vi "RF_SPW_Upsample.vi"(7 "Header In":T1={"header info"={"Header"="", "Head length"=0}, "A/D info"={"# rf points per line"=0, "# lines per scan"=0, "sample rate MHz"=0, "# A/D bits"=0, "# bytes per A/D"=0, "TGC Flag"=0, "A/D Type"=""}, "Tranducer Info"={"bandwidth"=0.0, "center freq"=0.0, "start freq"=0.0, "ID"=0}, "Scan Info"={"delay"=0.0, "pivot distance"=0.0, "sector scan angle"=0.0, "operator"="", "Scan Mode"="", "location"=""}, "Time/Date Info"={"date"="", "time"=""}, "RF Info"={"RF file name"="", "RF file att"="", "RF cal file name"="", "RF cal file att"=""}, "Patient Info"={"ID"="", "extended ID"="", "age"=0, "sex"="", "previously\nscanned"="", "PSA"=0.0, "LOS"=1, "Ethnicty 2"=3, "Race"=3}, "Tissue Type"={"organ"=0, "disease type"=0, "disease location"=0, "IQ_pts"=0, "RcvBuffer"=0, "RcvFrame"=0, "IQBuff"=0, "IQFrame"=0, "IQPage"=0}, "Votage scaling"={"Digitizer (dB)"=0.0, "Gain (dB)"=0.0, "Atten (dB)"=0.0}, "Comment"="", "Misc Info"={"avg num"=0, "c speed"=0, "Div By or SF zones"=0, "XMIT CHS"=0, "RCV CHS"=0, "Xmit angle"=0.0}, "Therapy Parameters"={"Theraputic Freq (MHz)"=0.1, "Time on (s)"=1.0, "Therapy amplitude (mV)"=50.0, "Lines Before"=20, "Lines After"=80}, "Scan Settings"={"Energy (uJ or V)"=0, "Damp (Ohm) or Fc"=0, "HP Filt (KHz)"=0, "LP Filt (MHz)"=0, "Gain (db)"=0, "prf (kHz)"=0.0, "Distance between\nscan lines (um)"=0, "Distance between\nscan planes (um)"=0, "Scan line gap (um)"=0.0, "Scan plane gap (um)"=0.0}, "Compression Parameters"={"F1 (MHz)"=0.0, "F2 (MHz)"=0.0, "% taper"=0.0, "duration"=0.0}, "Patient Info Xtra"={"First Name"="", "Last Name"="", "Notes"=""}, "ROI Box"=[]} {"Compression Parameters"."% taper" min=50 max=1000 format="%.2f"; "Compression Parameters"."F2 (MHz)" format="%.3f"; "Compression Parameters"."F1 (MHz)" format="%.3f"; "Scan Settings"."prf (kHz)" format="%.2f"; "Therapy Parameters"."Therapy amplitude (mV)" min=50 max=1000 format="%.2f"; "Therapy Parameters"."Time on (s)" format="%.3f"; "Therapy Parameters"."Theraputic Freq (MHz)" format="%.3f"; "Patient Info"."Race" items=["Am Ind or Alaska", "Asian", "Hawaiian, Pac Isl", "Black or Afr Amer", "White", "more than one race", "unknown"]; "Patient Info"."Ethnicty 2" items=["Hispanic", "Non-Hispanic", "unknown"]; "Patient Info"."LOS" items=["1", "2", "3", "4", "5"]; "Patient Info"."PSA" format="%.1f"; "Scan Info"."delay" format="%.2f"; "Scan Info"."pivot distance" format="%.2f"; "Scan Info"."sector scan angle" format="%.2f"; "Tranducer Info"."bandwidth" format="%.2f"; "Tranducer Info"."center freq" format="%.2f"; "Tranducer Info"."start freq" format="%.2f"}, 9 "RF Data In":i16[](array[numeric])) -> (0 "Header Out":T1={"header info"={"Header"="", "Head length"=0}, "A/D info"={"# rf points per line"=0, "# lines per scan"=0, "sample rate MHz"=0, "# A/D bits"=0, "# bytes per A/D"=0, "TGC Flag"=0, "A/D Type"=""}, "Tranducer Info"={"bandwidth"=0.0, "center freq"=0.0, "start freq"=0.0, "ID"=0}, "Scan Info"={"delay"=0.0, "pivot distance"=0.0, "sector scan angle"=0.0, "operator"="", "Scan Mode"="", "location"=""}, "Time/Date Info"={"date"="", "time"=""}, "RF Info"={"RF file name"="", "RF file att"="", "RF cal file name"="", "RF cal file att"=""}, "Patient Info"={"ID"="", "extended ID"="", "age"=0, "sex"="", "previously\nscanned"="", "PSA"=0.0, "LOS"=1, "Ethnicty 2"=3, "Race"=3}, "Tissue Type"={"organ"=0, "disease type"=0, "disease location"=0, "IQ_pts"=0, "RcvBuffer"=0, "RcvFrame"=0, "IQBuff"=0, "IQFrame"=0, "IQPage"=0}, "Votage scaling"={"Digitizer (dB)"=0.0, "Gain (dB)"=0.0, "Atten (dB)"=0.0}, "Comment"="", "Misc Info"={"avg num"=0, "c speed"=0, "Div By or SF zones"=0, "XMIT CHS"=0, "RCV CHS"=0, "Xmit angle"=0.0}, "Therapy Parameters"={"Theraputic Freq (MHz)"=0.0, "Time on (s)"=0.0, "Therapy amplitude (mV)"=0.0, "Lines Before"=0, "Lines After"=0}, "Scan Settings"={"Energy (uJ or V)"=0, "Damp (Ohm) or Fc"=0, "HP Filt (KHz)"=0, "LP Filt (MHz)"=0, "Gain (db)"=0, "prf (kHz)"=0.0, "Distance between\nscan lines (um)"=0, "Distance between\nscan planes (um)"=0, "Scan line gap (um)"=0.0, "Scan plane gap (um)"=0.0}, "Compression Parameters"={"F1 (MHz)"=0.0, "F2 (MHz)"=0.0, "% taper"=0.0, "duration"=0.0}, "Patient Info Xtra"={"First Name"="", "Last Name"="", "Notes"=""}, "ROI Box"=[0, 0, 0, 0]} {"Compression Parameters"."% taper" min=50 max=1000 format="%.2f"; "Compression Parameters"."F2 (MHz)" format="%.3f"; "Compression Parameters"."F1 (MHz)" format="%.3f"; "Scan Settings"."prf (kHz)" format="%.2f"; "Therapy Parameters"."Therapy amplitude (mV)" min=50 max=1000 format="%.2f"; "Therapy Parameters"."Time on (s)" format="%.3f"; "Therapy Parameters"."Theraputic Freq (MHz)" format="%.3f"; "Patient Info"."Race" items=["Am Ind or Alaska", "Asian", "Hawaiian, Pac Isl", "Black or Afr Amer", "White", "more than one race", "unknown"]; "Patient Info"."Ethnicty 2" items=["Hispanic", "Non-Hispanic", "unknown"]; "Patient Info"."LOS" items=["1", "2", "3", "4", "5"]; "Patient Info"."PSA" format="%.1f"; "Scan Info"."delay" format="%.2f"; "Scan Info"."pivot distance" format="%.2f"; "Scan Info"."sector scan angle" format="%.2f"; "Tranducer Info"."bandwidth" format="%.2f"; "Tranducer Info"."center freq" format="%.2f"; "Tranducer Info"."start freq" format="%.2f"}, 1 "RF Out 2D":i16[][](graph), 2 "RF pts out":i32, 3 "RF Array Out":i16[](array[numeric]))   [LabVIEW 2022 SP3]
uses:
  ViewData/-ReadEye/Header.ctl
  <vilib>/Analysis/1siggen.llb/Ramp Pattern by Samples.vi
  <vilib>/gmath/NI_Gmath.lvlib
  <vilib>/Analysis/NI_AALBase.lvlib
panel:
  out "RF 2D in":i16[][](graph)
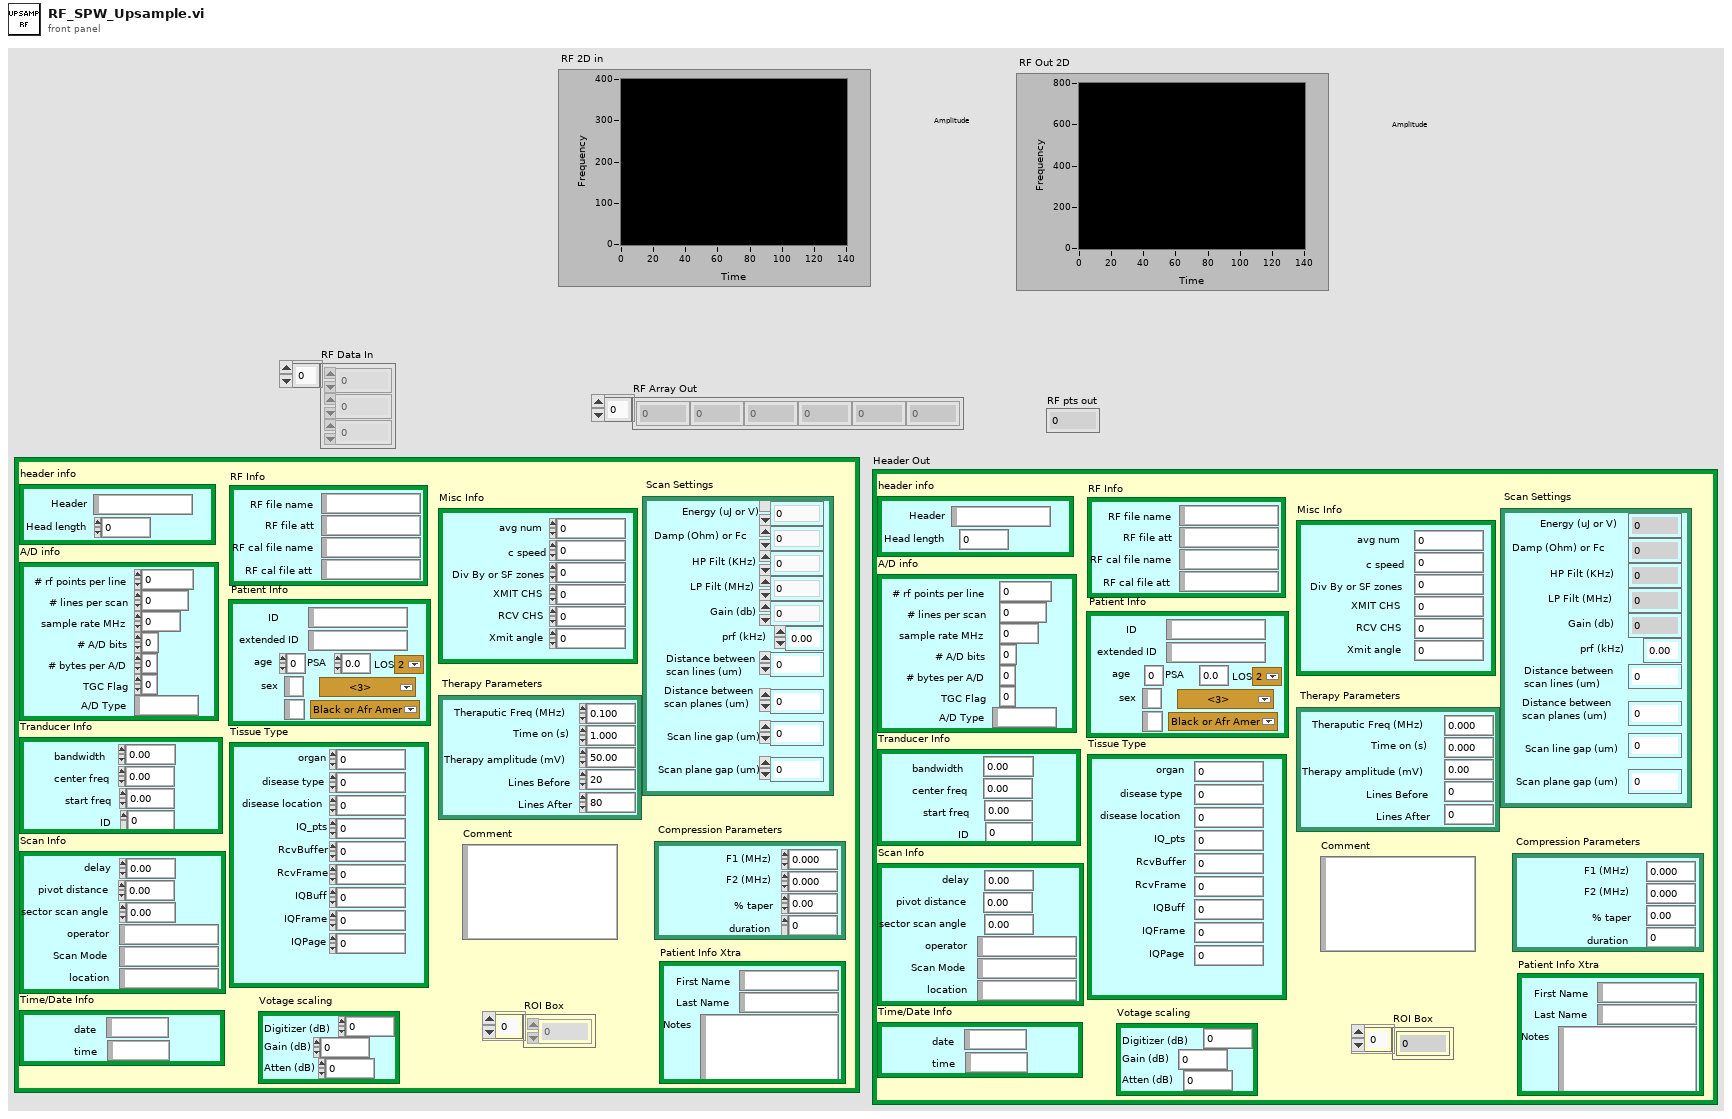
[diagram p1: front panel]
types:
  T1 = typedef "Header.ctl" = cluster{"header info":cluster{"Header":string, "Head length":i16}, "A/D info":cluster{"# rf points per line":u16, "# lines per scan":u16, "sample rate MHz":u16, "# A/D bits":i16, "# bytes per A/D":u16, "TGC Flag":u16, "A/D Type":string}, "Tranducer Info":cluster{"bandwidth":sgl, "center freq":sgl, "start freq":sgl, "ID":i32}, "Scan Info":cluster{"delay":sgl, "pivot distance":sgl, "sector scan angle":sgl, "operator":string, "Scan Mode":string, "location":string}, "Time/Date Info":cluster{"date":string, "time":string}, "RF Info":cluster{"RF file name":string, "RF file att":string, "RF cal file name":string, "RF cal file att":string}, "Patient Info":cluster{"ID":string, "extended ID":string, "age":u16, "sex":string, "previously\nscanned":string, "PSA":sgl, "LOS":u8, "Ethnicty 2":u8, "Race":u8}, "Tissue Type":cluster{"organ":i16, "disease type":i16, "disease location":i16, "IQ_pts":u16, "RcvBuffer":u8, "RcvFrame":u16, "IQBuff":u8, "IQFrame":u16, "IQPage":u8}, "Votage scaling":cluster{"Digitizer (dB)":sgl, "Gain (dB)":sgl, "Atten (dB)":sgl}, "Comment":string, "Misc Info":cluster{"avg num":u16, "c speed":i16, "Div By or SF zones":i16, "XMIT CHS":u8, "RCV CHS":u8, "Xmit angle":sgl}, "Therapy Parameters":cluster{"Theraputic Freq (MHz)":sgl, "Time on (s)":sgl, "Therapy amplitude (mV)":sgl, "Lines Before":u16, "Lines After":u16}, "Scan Settings":cluster{"Energy (uJ or V)":u8, "Damp (Ohm) or Fc":u8, "HP Filt (KHz)":u8, "LP Filt (MHz)":u8, "Gain (db)":u8, "prf (kHz)":sgl, "Distance between\nscan lines (um)":u16, "Distance between\nscan planes (um)":u16, "Scan line gap (um)":sgl, "Scan plane gap (um)":sgl}, "Compression Parameters":cluster{"F1 (MHz)":sgl, "F2 (MHz)":sgl, "% taper":sgl, "duration":sgl}, "Patient Info Xtra":cluster{"First Name":string, "Last Name":string, "Notes":string}, "ROI Box":u16[]}
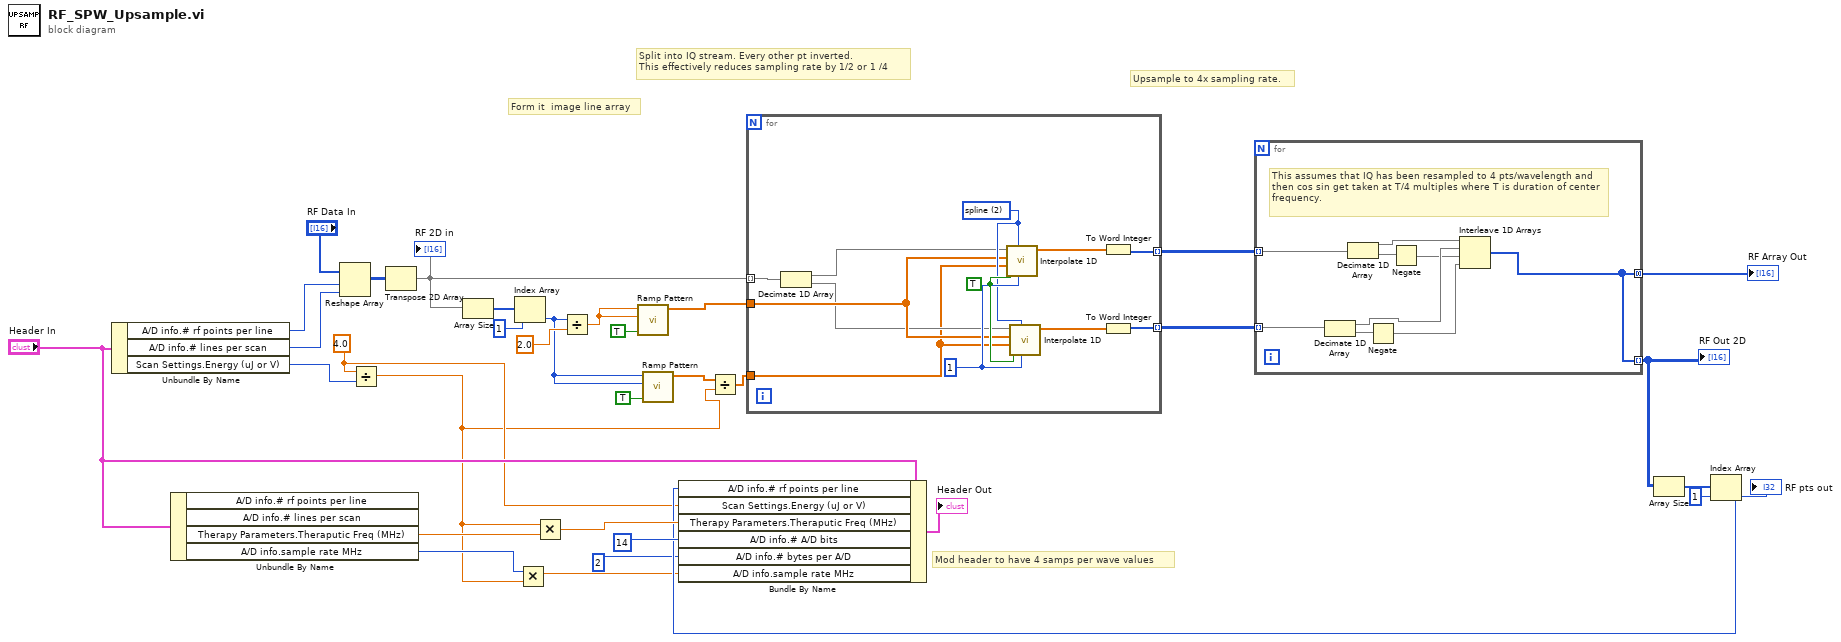
[diagram p0: block diagram]
diagram:
  w2 = sgl 4.0 ("value")
  # "Mod header to have 4 samps per wave values"
  # "Upsample to 4x sampling rate."
  # "Form it  image line array"
  # "Split into IQ stream. Every other pt inverted.\nThis effectively reduces sampling rate by 1/2 or 1 /4"
  n1 = Unbundle By Name("Header In") -> ("A/D info.# rf points per line"=w26:u16, "A/D info.# lines per scan"=w27:u16, "Scan Settings.Energy (uJ or V)"=w33:u8)
  n2 = Unbundle By Name("Header In") -> ("Therapy Parameters.Theraputic Freq (MHz)"=w31:sgl, "A/D info.sample rate MHz"=w4:u16)  [unwired: 2 out]
  n3 = Reshape Array("RF Data In", w26, w27) -> (w28:i16[][])
  n4 = Divide(x=w2, y=w33) -> (x/y=w1:sgl)
  n5 = Transpose 2D Array(2D array=w28) -> (transposed array=w16:i16[][])
  "RF 2D in" <- w16
  n6 = Array Size(array=w16) -> (size(s)=w23:i32[])
  n7 = Index Array(array=w23, index=1) -> (element=w8:i32)
  n8 = Multiply(x=w4, y=w1) -> (x*y=w3:sgl)
  n9 = Multiply(x=w1, y=w31) -> (x*y=w30:sgl)
  n10 = Divide(x=w8, y=sgl 2.0 ("value")) -> (x/y=w19:sgl)
  n11 = call-poly <vilib>:"Ramp Pattern.vi"("exclude end?"=TRUE, "end"=w19, "samples"=w19) -> ("Ramp Pattern"=w17:dbl[])  [unwired: 7 in, 1 out]
  n12 = call-poly <vilib>:"Ramp Pattern.vi"("exclude end?"=TRUE, "end"=w8, "samples"=w8) -> ("Ramp Pattern"=w7:dbl[])  [unwired: 7 in, 1 out]
  n13 = Divide(x=w7, y=w1) -> (x/y=w6:dbl[])
  n14 = for {
    tunnel: [w44] -> w25 mode=indexing
    tunnel: [w45] -> w24 mode=indexing
    tunnel: w16 -> [w35] mode=indexing
    tunnel: w17 -> [w40]
    tunnel: w6 -> [w34]
    w43 = 1 ("ntimes")
    w42 = TRUE ("X is monotonic")
    w41 = 2 items=["nearest", "linear", "spline", "cubic Hermite", "Lagrange"] ("method")
    n15 = Decimate 1D Array(w35) -> (w39:i16[], w38:i16[])
    n16 = call <vilib>:"Interpolate 1D.vi"("ntimes"=w43, "method"=w41, "X is monotonic"=w42, "xi"=w34, "X"=w40, "Y"=w39) -> ("yi"=w37:dbl[])  [unwired: 3 in, 2 out]
    n17 = call <vilib>:"Interpolate 1D.vi"("ntimes"=w43, "method"=w41, "X is monotonic"=w42, "xi"=w34, "X"=w40, "Y"=w38) -> ("yi"=w36:dbl[])  [unwired: 3 in, 2 out]
    n18 = To Word Integer(number=w37) -> (16bit integer=w44:i16[])
    n19 = To Word Integer(number=w36) -> (16bit integer=w45:i16[])
  }
  n20 = for {
    tunnel: [w46] -> w18 mode=concatenating
    tunnel: w25 -> [w54] mode=indexing
    tunnel: w24 -> [w53] mode=indexing
    tunnel: [w46] -> w15 mode=indexing
    # "This assumes that IQ has been resampled to 4 pts/wavelength and then cos sin get taken at T/4 multiples where T is duration of center frequency."
    n21 = Decimate 1D Array(w53) -> (w49:i16[], w51:i16[])
    n22 = Decimate 1D Array(w54) -> (w50:i16[], w52:i16[])
    n23 = Negate(x=w51) -> (-x=w47:i16[])
    n24 = Negate(x=w52) -> (-x=w48:i16[])
    n25 = Interleave 1D Arrays(w50, w49, w48, w47) -> (w46:i16[])
  }
  "RF Array Out" <- w18
  "RF Out 2D" <- w15
  n26 = Array Size(array=w15) -> (size(s)=w14:i32[])
  n27 = Index Array(array=w14, index=1) -> (element=w11:i32)
  "RF pts out" <- w11
  n28 = Bundle By Name(cluster="Header In", "A/D info.# rf points per line"=w11, "Scan Settings.Energy (uJ or V)"=w2, "Therapy Parameters.Theraputic Freq (MHz)"=w30, "A/D info.# A/D bits"=i16 14, "A/D info.# bytes per A/D"=i16 2 ("A/D info.# A/D bits"), "A/D info.sample rate MHz"=w3) -> (→"Header Out":T1)
